vi "Coerse row column.vi"(3 "Row Col":i32, 4 "Board Size":i32) -> (5 "Coerced Out":i32)   [LabVIEW 2017, in "AntFarm_MB.lvclass"]
uses:
  AntFarm_MB.lvclass
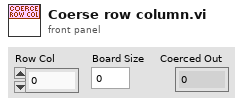
[diagram p1: front panel]
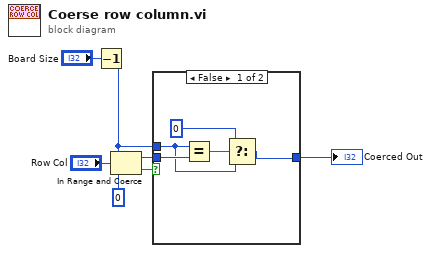
[diagram p0: block diagram]
diagram:
  n1 = Decrement(x="Board Size") -> (x-1=w7:i32)
  n2 = In Range and Coerce(upper limit=w7, x="Row Col", lower limit=0) -> (coerced(x)=w5:i32, In Range?=w4:bool)
  n3 = case shown="False" w4 {
    tunnel: w5 -> [w12 w13]
    tunnel: [w8 w13] -> w6
    tunnel: w7 -> [w9 _]
    frame False {
      n4 = Equal?(x=w9, y=w12) -> (x = y?=w11:bool)
      n5 = Select(t=0, s=w11, f=w9) -> (s? t:f=w8:i32)
    }
    frame True {
    }
  }
  "Coerced Out" <- w6
